vi "GEOM_GetValsFromSection.vi"(10 "section":string) -> (0 "yend":i32, 1 "ystart":i32, 2 "xend":i32, 3 "xstart":i32, 4 "ye str":string, 5 "xe str":string, 6 "ys str":string, 7 "xs str":string)   [LabVIEW 2016]
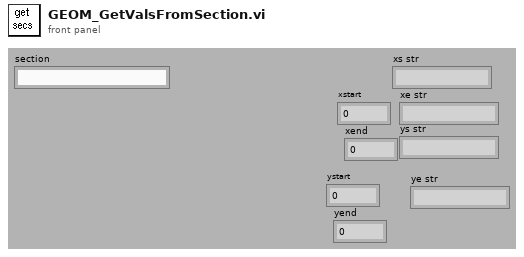
[diagram p1: front panel]
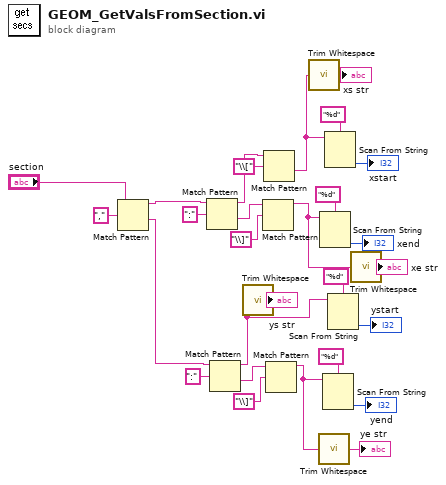
[diagram p0: block diagram]
diagram:
  n1 = Match Pattern(string="section", regular expression=",") -> (before substring=w26:string, after substring=w6:string)  [unwired: 3 out]
  n2 = Match Pattern(string=w26, regular expression=":") -> (before substring=w21:string, after substring=w25:string)  [unwired: 3 out]
  n3 = Match Pattern(string=w6, regular expression=":") -> (before substring=w5:string, after substring=w8:string)  [unwired: 3 out]
  n4 = call <vilib>:"Trim Whitespace.vi"("string"=w5) -> ("trimmed string"=→"ys str":string)  [unwired: 1 in]
  n5 = Match Pattern(string=w25, regular expression="\\]") -> (before substring=w23:string)  [unwired: 4 out]
  n6 = Match Pattern(string=w21, regular expression="\\[") -> (after substring=w16:string)  [unwired: 4 out]
  n7 = Match Pattern(string=w8, regular expression="\\]") -> (before substring=w10:string)  [unwired: 4 out]
  n8 = call <vilib>:"Trim Whitespace.vi"("string"=w16) -> ("trimmed string"=→"xs str":string)  [unwired: 1 in]
  n9 = call <vilib>:"Trim Whitespace.vi"("string"=w10) -> ("trimmed string"=→"ye str":string)  [unwired: 1 in]
  n10 = Scan From String(format string="%d", input string=w23) -> (output 1=→"xend":i32)  [unwired: 2 in, 4 out]
  n11 = Scan From String(format string="%d", input string=w10) -> (output 1=→"yend":i32)  [unwired: 2 in, 4 out]
  n12 = Scan From String(format string="%d", input string=w16) -> (output 1=→"xstart":i32)  [unwired: 2 in, 4 out]
  n13 = Scan From String(format string="%d", input string=w5) -> (output 1=→"ystart":i32)  [unwired: 2 in, 4 out]
  n14 = call <vilib>:"Trim Whitespace.vi"("string"=w23) -> ("trimmed string"=→"xe str":string)  [unwired: 1 in]
